vi "Pre Launch Init.vi"(11 "Logged Actor in":refnum<class "LoggedActor.lvclass">) -> (0 "error out":errorcluster, 3 "Logged Actor out":refnum<class "LoggedActor.lvclass">)   [LabVIEW 2020, in "LoggedActor.lvclass"]
doc: "(<B>Filename</B>: Actor Framework.lvlib:Actor.lvclass:Pre Launch Init.vi)\n\nDefines behavior that occurs after the Launch Nested Actor method is invoked but before the actor's Actor Core method begins running.\n\nBy default, this method does nothing. A descendant class may override it to define behavior."
uses:
  <vilib>/gpm_packages/@cs/Network-interface/Source/Logged Actor/LoggedActor.lvclass
  C:/Program Files/National Instruments/LabVIEW 2020/vi.lib/ActorFramework/Actor/Actor.lvclass
  <vilib>/gpm_packages/@cs/event-logger/Source/Composed Log/Types/Log Level.ctl
  <vilib>/gpm_packages/@cs/Network-interface/Source/Logged Actor/LoggedActor.lvclass/LoggedActor.ctl
  <vilib>/ActorFramework/Actor/Actor.lvclass/Actor.ctl
  <vilib>/ActorFramework/Message Enqueuer/Message Enqueuer.lvclass/Message Enqueuer.ctl
  <vilib>/gpm_packages/@cs/event-logger/Source/Composed Log/LoggerReference/LoggerReference.lvclass/LoggerReference.ctl
  <vilib>/gpm_packages/@cs/event-logger/Source/Composed Log/LoggerReference/Log Event.vi
  <vilib>/ActorFramework/Message Enqueuer/Init from Existing Queue.vi
  <vilib>/gpm_packages/@cs/event-logger/Source/Composed Log/LoggerReference/Log.vi
  <vilib>/gpm_packages/@cs/event-logger/Source/Composed Log/LoggerReference/Get Valid Event Time.vi
  <vilib>/gpm_packages/@cs/event-logger/Source/Composed Log/LoggerReference/Remove Stale Logs.vi
  <vilib>/ActorFramework/Actor/Actor.lvclass
  <vilib>/ActorFramework/Message Enqueuer/Message Enqueuer.lvclass
  <vilib>/gpm_packages/@cs/event-logger/Source/Composed Log/Composed Log.lvlib
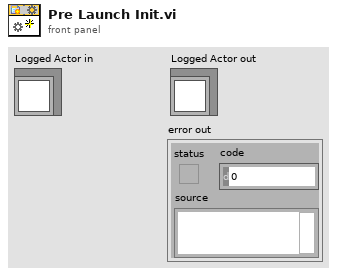
[diagram p1: front panel]
types:
  T1 = typedef "Composed Log.lvlib/Log Level.ctl" = enum16{"Debug", "Info", "Warning", "Error", "Critical"}
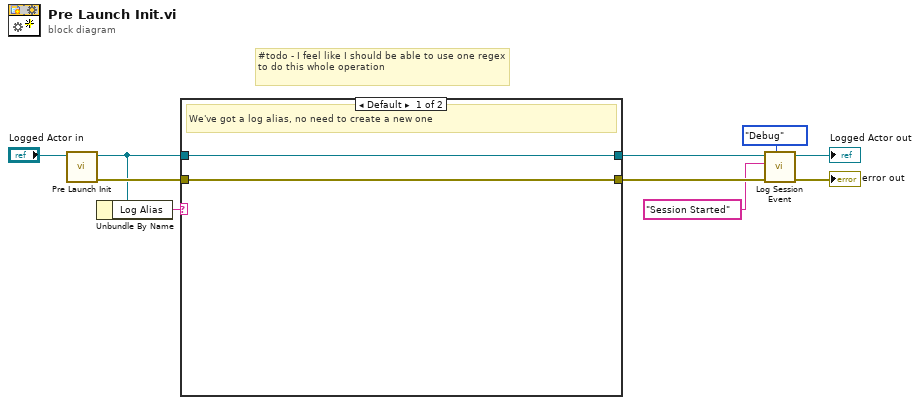
[diagram p0: block diagram]
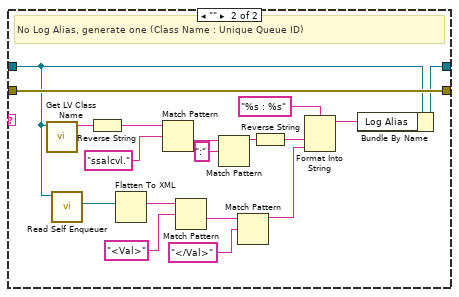
[diagram p2: hidden frame]
diagram:
  # "#todo - I feel like I should be able to use one regex to do this whole operation"
  n1 = call-parent "Pre Launch Init.vi"("Actor in"="Logged Actor in") -> ("error out"=w5:errorcluster, "Actor out"=w3:refnum<class "LoggedActor.lvclass">)  [unwired: 9 in]
  n2 = Unbundle By Name(w3) -> ("Log Alias"=w2:string)
  n3 = case shown="Default" w2 {
    tunnel: w3 -> [w12 w14]
    tunnel: [w12 w23] -> w6
    tunnel: w5 -> [w11 w24]
    tunnel: [w11 w24] -> w4
    frame Default {
      # "We've got a log alias, no need to create a new one"
    }
    frame "" {
      # "No Log Alias, generate one (Class Name : Unique Queue ID)"
      n4 = call <vilib>:"Get LV Class Name.vi"("object"=w14) -> ("class name"=w30:string)  [unwired: 9 in, 1 out]
      n5 = call <vilib>:"Read Self Enqueuer.vi"("Actor"=w14) -> ("Self Enqueuer"=w13:refnum<class "Message Enqueuer.lvclass">)  [unwired: 10 in]
      n6 = Reverse String(1:w30) -> (0:w29:string)
      n7 = Flatten To XML(6:w13) -> (2:w19:string)
      n8 = Match Pattern(string=w29, regular expression="ssalcvl.") -> (after substring=w27:string)  [unwired: 1 in, 3 out]
      n9 = Match Pattern(string=w19, regular expression="<Val>") -> (after substring=w17:string)  [unwired: 1 in, 3 out]
      n10 = Match Pattern(string=w27, regular expression=":") -> (before substring=w25:string)  [unwired: 1 in, 3 out]
      n11 = Match Pattern(string=w17, regular expression="</Val>") -> (before substring=w15:string)  [unwired: 1 in, 3 out]
      n12 = Reverse String(1:w25) -> (0:w22:string)
      n13 = Format Into String(format string="%s : %s", w22, w15) -> (resulting string=w21:string)  [unwired: 2 in, 1 out]
      n14 = Bundle By Name(cluster=w14, "Log Alias"=w21) -> (w23:refnum<class "LoggedActor.lvclass">)
    }
  }
  n15 = call <vilib>:"Log Session Event.vi"("Event Level"=Log_Level."Debug", "error in (no error)"=w4, "Event Data"="Session Started", "SessionActor in"=w6) -> ("error out"=→"error out":errorcluster, "SessionActor out"=→"Logged Actor out":refnum<class "LoggedActor.lvclass">)  [unwired: 6 in]
